vi "Serial Read to CRLF.vi"(8 "error in":errorcluster, 9 "timeout (ms)":i32, 10 "bytes to read":u32, 11 "Visa Resource":refnum<visa-resource-name>) -> (0 "error out":errorcluster, 1 "timed out?":bool, 3 "data":u8[](array[numeric]))   [LabVIEW 2013, in "Serial Shared Components.lvlib"]
doc: "Performs a read on the serial port."
uses:
  Serial Shared Components.lvlib
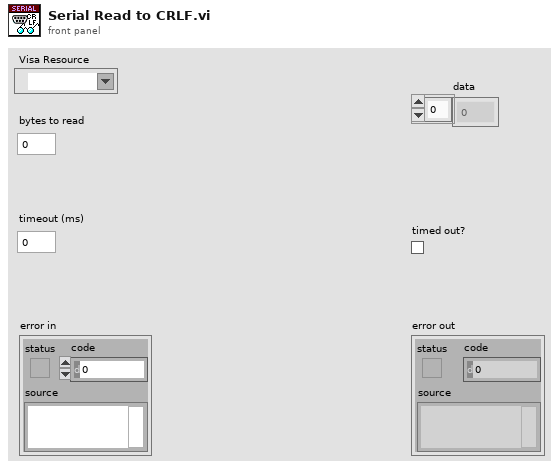
[diagram p1: front panel]
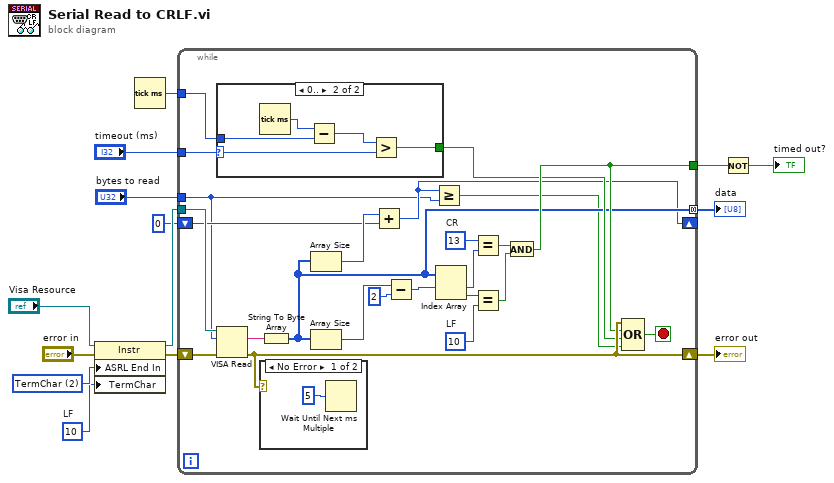
[diagram p0: block diagram]
diagram:
  w5 = u8 10  # LF
  w6 = u16 2 items=["None", "Last Bit", "TermChar"] ("Serial Settings:End Mode for Reads")
  n1 = property class="Instr"(reference="Visa Resource", error in="error in", "ASRL End In"=w6, "TermChar"=w5) -> (reference out=w7:refnum<visa-resource-name>, error out=w9:errorcluster)
  n2 = Tick Count (ms)() -> (millisecond timer value=w4:u32)
  n3 = while {
    tunnel: w4 -> [w36]
    shift-right: [w34] -> w11
    shift-left: w9 -> [w38]
    tunnel: "bytes to read" -> [w16]
    tunnel: w7 -> [w35]
    tunnel: [w23] -> w3
    tunnel: "timeout (ms)" -> [w21]
    tunnel: [w20] -> w2 mode=concatenating
    shift-right: [w17] -> _
    shift-left: 0 -> [w18]
    stop <- w37 stop-if-true
    w26 = u8 10  # LF
    w27 = u8 13  # CR
    n4 = case shown="0.." w21 {
      selector: w21 -> [_ w39]
      tunnel: w36 -> [_ w42]
      tunnel: [_ w40] -> w22
      frame ..-1 {
        # "no t/o"
      }
      frame 0.. {
        n5 = Tick Count (ms)() -> (millisecond timer value=w43:u32)
        n6 = Subtract(x=w43, y=w42) -> (x-y=w41:u32)
        n7 = Greater?(x=w41, y=w39) -> (0:w40:bool)
      }
    }
    n8 = VISA Read(VISA resource name=w35, byte count=w16, error in (no error)=w38) -> (read buffer=w33:string, error out=w34:errorcluster)  [unwired: 2 out]
    n9 = case shown="No Error" w34 {
      frame No Error {
        n10 = Wait Until Next ms Multiple(millisecond multiple=u32 5) -> ()  [unwired: 1 out]
      }
      frame Error {
      }
    }
    n11 = String To Byte Array(string=w33) -> (unsigned byte array=w20:u8[])
    n12 = Array Size(array=w20) -> (size(s)=w19:i32)
    n13 = Array Size(array=w20) -> (size(s)=w32:i32)
    n14 = Add(x=w19, y=w18) -> (x+y=w17:i32)
    n15 = Subtract(x=w32, y=2) -> (x-y=w30:i32)
    n16 = Greater Or Equal?(x=w17, y=w16) -> (x >= y?=w15:bool)
    n17 = Index Array(array=w20, index #1=w30) -> (element #1=w29:u8, element #2=w28:u8)  [unwired: 1 in]
    n18 = Equal?(x=w27, y=w29) -> (x = y?=w24:bool)
    n19 = Equal?(x=w28, y=w26) -> (x = y?=w25:bool)
    n20 = And(x=w24, y=w25) -> (x .and. y?=w23:bool)
    n21 = Compound Arithmetic op=OR(w34, w23, w22, w15) -> (w37:bool)
  }
  "error out" <- w11
  "data" <- w2
  n22 = Not(x=w3) -> (.not. x?=→"timed out?":bool)
